vi "Get Active Project.vi"(11 "error in":errorcluster) -> (4 "path":path, 6 "name":string, 15 "error out":errorcluster)   [LabVIEW 2021, in "InstrumentStudio Plug-In Editor.lvlib"]
uses:
  InstrumentStudio Plug-In Editor.lvlib
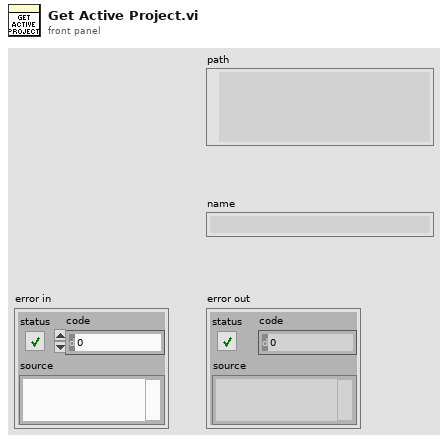
[diagram p1: front panel]
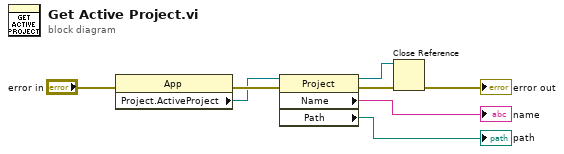
[diagram p0: block diagram]
diagram:
  n1 = property class="App"(error in="error in") -> (error out=w7:errorcluster, "Project.ActiveProject"=w1:refnum<vi>)  [unwired: 1 in, 1 out]
  n2 = property class="Project"(reference=w1, error in=w7) -> (reference out=w2:refnum<vi>, error out=w6:errorcluster, "Name"=→"name":string, "Path"=→"path":path)
  n3 = Close Reference(reference=w2, error in (no error)=w6) -> (error out=→"error out":errorcluster)
